vi "Inverse Kinematics.vi"(8 "Radii (ft)":T4 {"Right Back Position" format="%.2f"; "Right Front Position" format="%.2f"; "Left Back Position" format="%.2f"; "Left Front Position" format="%.2f"}, 11 "Target Velocity (ft/s and deg/s)":T1) -> (2 "Pod Setpoints (ft/s and deg)":T2, 4 "cross products":T3, 6 "translation":dbl[](array[numeric]))   [LabVIEW 2025]
doc: "This VI calculates the velocity setpoints needed for the pods of a Swerve Drive. It takes in Robot centric velocities that describe the robot's motion, a cluster of the current orientations in degrees of each of the pods, and a cluster of the radius vectors from the center of mass to each of the swerve pods. It then outputs four clusters that represent the pod setpoints (velocity of the pod and orientation of the pod in ft/s and deg/s)\n\nOrder of all the clusters holding some kind of pod information will always be Left Front, Left Back, Right Front, Right Back"
uses:
  Type Definitions/Data/Pod Positions.ctl
  Type Definitions/Data/Pod Setpoints.ctl
  Type Definitions/Data/Robot Velocities.ctl
  <vilib>/Analysis/coordinate.llb/Angle Units.ctl
  <vilib>/Analysis/coordinate.llb/Angle Range (Degree).ctl
  <vilib>/Analysis/coordinate.llb/Wrap Angle (scalar).vi
  <vilib>/Analysis/_algsub.llb/Real Vector Norm.vi
  <vilib>/Analysis/NI_AALPro.lvlib
  <vilib>/Analysis/NI_AAL_Angle.lvlib
panel:
  # "Diganostics for the Visualizer"
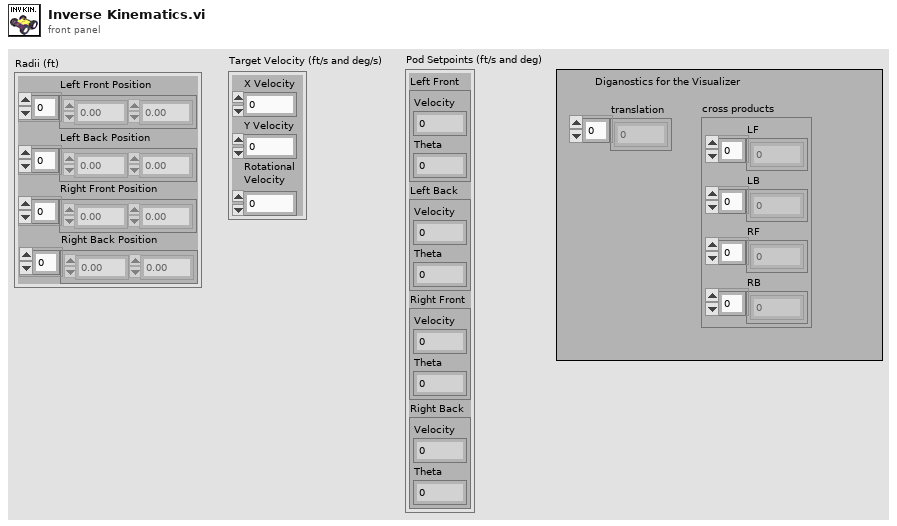
[diagram p1: front panel]
types:
  T1 = typedef "Robot Velocities.ctl" = cluster{"X Velocity":dbl, "Y Velocity":dbl, "Rotational \nVelocity":dbl}
  T2 = typedef "Pod Setpoints.ctl" = cluster{"Left Front":cluster{"Velocity":dbl, "Theta":dbl}, "Left Back":cluster{"Velocity":dbl, "Theta":dbl}, "Right Front":cluster{"Velocity":dbl, "Theta":dbl}, "Right Back":cluster{"Velocity":dbl, "Theta":dbl}}
  T3 = cluster{"LF":dbl[], "LB":dbl[], "RF":dbl[], "RB":dbl[]}
  T4 = typedef "Pod Positions.ctl" = cluster{"Left Front Position":dbl[], "Left Back Position":dbl[], "Right Front Position":dbl[], "Right Back Position":dbl[]}
  T5 = typedef "NI_AAL_Angle.lvlib/Angle Range (Degree).ctl" = u16
  T6 = typedef "NI_AAL_Angle.lvlib/Angle Units.ctl" = i32
  T7 = cluster{"[0]":cluster{"Velocity":dbl, "Theta":dbl}, "[1]":cluster{"Velocity":dbl, "Theta":dbl}, "[2]":cluster{"Velocity":dbl, "Theta":dbl}, "[3]":cluster{"Velocity":dbl, "Theta":dbl}}
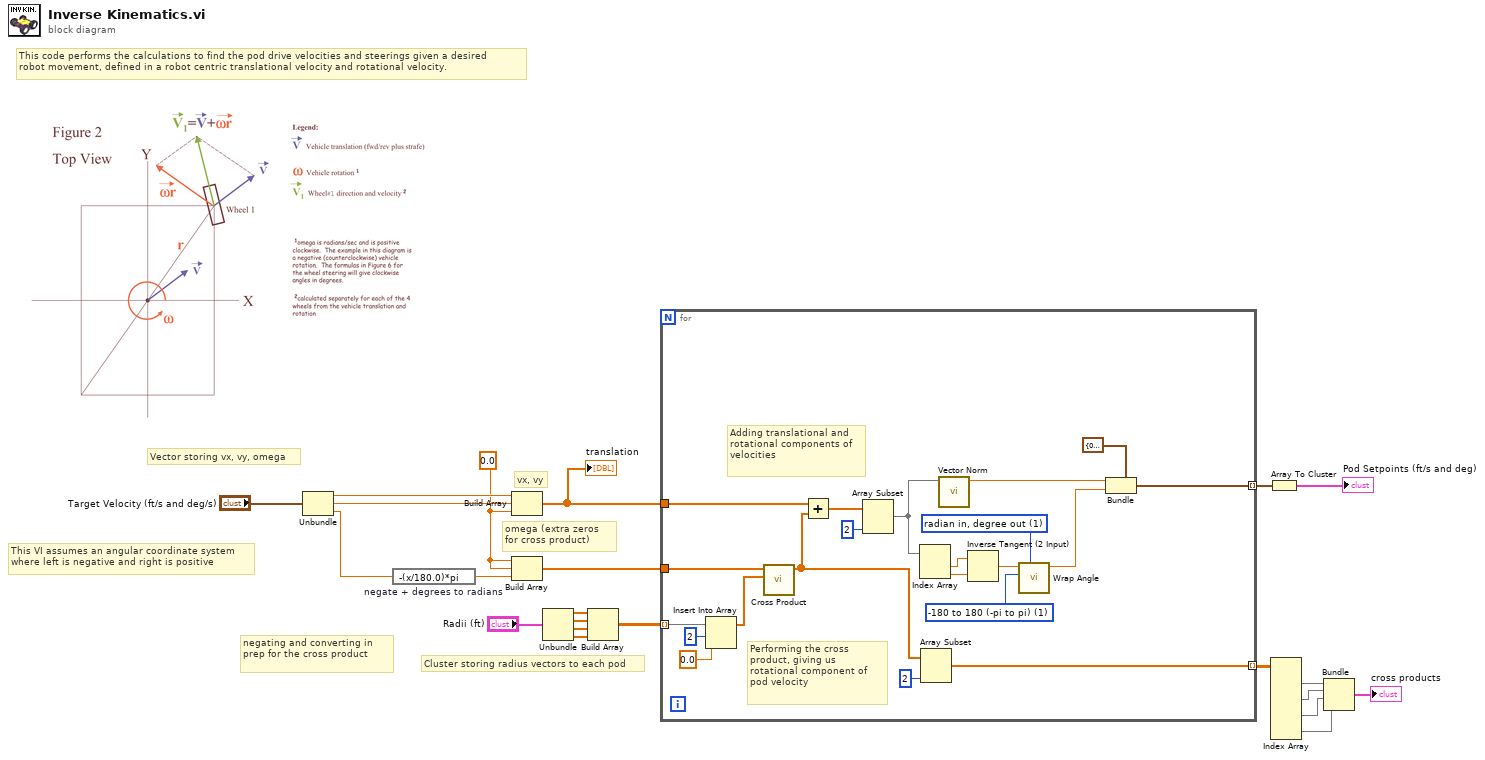
[diagram p0: block diagram]
diagram:
  w12 = 0.0 ("element")
  # "omega (extra zeros for cross product)"
  # "vx, vy"
  # "negating and converting in prep for the cross product"
  # "This code performs the calculations to find the pod drive velocities and steerings given a desired\nrobot movement, defined in a robot centric translational velocity and rotational velocity."
  # "This VI assumes an angular coordinate system\nwhere left is negative and right is positive"
  # "Cluster storing radius vectors to each pod"
  # "Vector storing vx, vy, omega"
  n1 = Unbundle("Target Velocity (ft/s and deg/s)") -> ("X Velocity"=w14:dbl, "Y Velocity"=w13:dbl, "Rotational \nVelocity"=w20:dbl)
  n2 = expression code="-(x/180.0)*pi" "negate + degrees to radians"(w20) -> (w11:dbl)
  n3 = Build Array(w14, w13, w12) -> (w8:dbl[])
  "translation" <- w8
  n4 = Build Array(w12, w12, w11) -> (w10:dbl[])
  n5 = Unbundle("Radii (ft)") -> ("Left Front Position"=w19:dbl[], "Left Back Position"=w18:dbl[], "Right Front Position"=w17:dbl[], "Right Back Position"=w16:dbl[])
  n6 = Build Array(w19, w18, w17, w16) -> (w15:dbl[][])
  n7 = for {
    tunnel: w15 -> [w43] mode=indexing
    tunnel: w8 -> [w40]
    tunnel: w10 -> [w39]
    tunnel: [w23] -> w9 mode=indexing
    tunnel: [w24] -> w7 mode=indexing
    w30 = T5 1 items=["none", "-180 to 180 (-pi to pi)", "0 to 360 (0 to 2pi)"] ("angle range")
    w31 = T6 1 items=["radian in, radian out", "radian in, degree out", "degree in, degree out", "degree in, radian out"] ("angle units")
    # "Performing the cross product, giving us\nrotational component of pod velocity"
    # "Adding translational and rotational components of velocities"
    n8 = Insert Into Array(array=w43, index=2, new element=0.0 ("new element/subarray")) -> (w38:dbl[])
    n9 = call <vilib>:"Cross Product.vi"("B Vector"=w38, "A Vector"=w39) -> ("Cross Product"=w26:dbl[])  [unwired: 8 in, 1 out]
    n10 = Add(x=w40, y=w26) -> (x+y=w37:dbl[])
    n11 = Array Subset(array=w37, length=2) -> (w35:dbl[])  [unwired: 1 in]
    n12 = Index Array(array=w35) -> (element #1=w34:dbl, element #2=w33:dbl)  [unwired: 2 in]
    n13 = Array Subset(array=w26, length=2) -> (w24:dbl[])  [unwired: 1 in]
    n14 = call-poly <vilib>:"Vector Norm.vi"("Input Vector"=w35) -> ("norm"=w29:dbl)  [unwired: 9 in, 1 out]
    n15 = Inverse Tangent (2 Input)(1:w33, 2:w34) -> (0:w32:dbl)
    n16 = call-poly <vilib>:"Wrap Angle.vi"("angle units"=w31, "angle range"=w30, "angle in"=w32) -> ("angle out"=w28:dbl)  [unwired: 7 in, 1 out]
    n17 = Bundle(cluster=cluster{"Velocity":dbl, "Theta":dbl} {"Velocity"=0.0, "Theta"=0.0} ("Pod Setpoints"), "Velocity"=w29, "Theta"=w28) -> (w23:cluster{"Velocity":dbl, "Theta":dbl})
  }
  n18 = Array To Cluster(array=w9) -> (cluster=→"Pod Setpoints (ft/s and deg)":T7)
  n19 = Index Array(array=w7) -> (element #1=w6:dbl[], element #2=w5:dbl[], element #3=w4:dbl[], element #4=w3:dbl[])  [unwired: 8 in]
  n20 = Bundle(w6, w5, w4, w3) -> (→"cross products":cluster{dbl[], dbl[], dbl[], dbl[]})  [unwired: 1 in]
